vi "To String.vi"(8 "error in (no error)":errorcluster, 11 "Acquired Result in":refnum<class "Acquired Result.lvclass">) -> (0 "error out":errorcluster, 2 "String":string, 3 "Acquired Result out":refnum<class "Acquired Result.lvclass">)   [LabVIEW 2019, in "Acquired Result.lvclass"]
uses:
  Acquired Result.lvclass
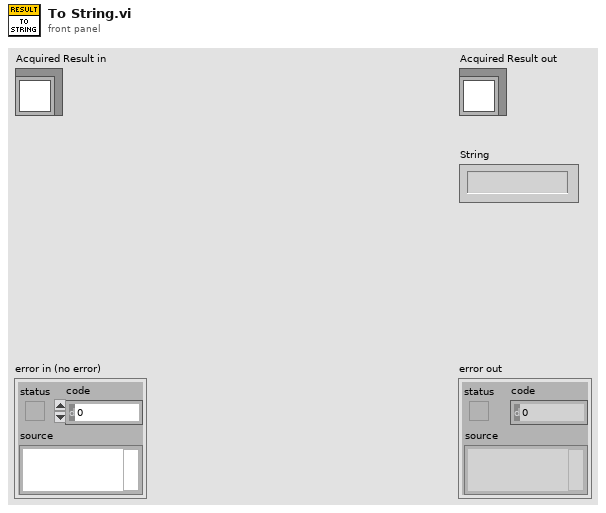
[diagram p1: front panel]
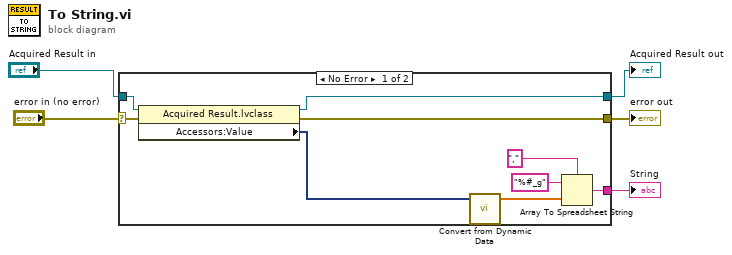
[diagram p0: block diagram]
diagram:
  n1 = case shown="No Error" "error in (no error)" {
    selector: "error in (no error)" -> [w14 w16]
    tunnel: [w13 w16] -> w4
    tunnel: [w11 w15] -> w2
    tunnel: "Acquired Result in" -> [w12 w15]
    tunnel: [w6 _] -> w1
    frame No Error {
      n2 = property class="Acquired Result.lvclass"(reference=w12, error in=w14) -> (reference out=w11:refnum<class "Acquired Result.lvclass">, error out=w13:errorcluster, "Accessors:Value"=w7:dynamicdata)
      n3 = call "Convert from Dynamic Data"("Dynamic Data Type"=w7) -> ("Array"=w10:dbl[])  [unwired: 3 in]
      n4 = Array To Spreadsheet String(delimiter (Tab)=",", array=w10, 3:"%#_g" ("format string")) -> (spreadsheet string=w6:string)
    }
    frame Error {
    }
  }
  "error out" <- w4
  "Acquired Result out" <- w2
  "String" <- w1
